vi "Log Data.vi"(0 "Test Inputs":T2 {"Nominal Output Voltage in V" format="%#.5g"; "Load Current in A" format="%#.5g"}, 5 "Test Results":T1 {"Measured Input Voltage in V" format="%#.5g"; "Dropout Voltage in V" format="%#.5g"; "Measured Output Voltage in V" format="%#.5g"}, 7 "DataLogger File Path":path, 11 "error in (no error)":errorcluster) -> (15 "error out":errorcluster)   [LabVIEW 2020, in "LDO Dropout Voltage.lvlib"]
uses:
  LDO Dropout Voltage.lvlib
  Typedefs/Test Inputs.ctl
  Typedefs/Advance Settings.ctl
  Reusables/Instrument APIs/Load Output Function.ctl
  Typedefs/Test Results.ctl
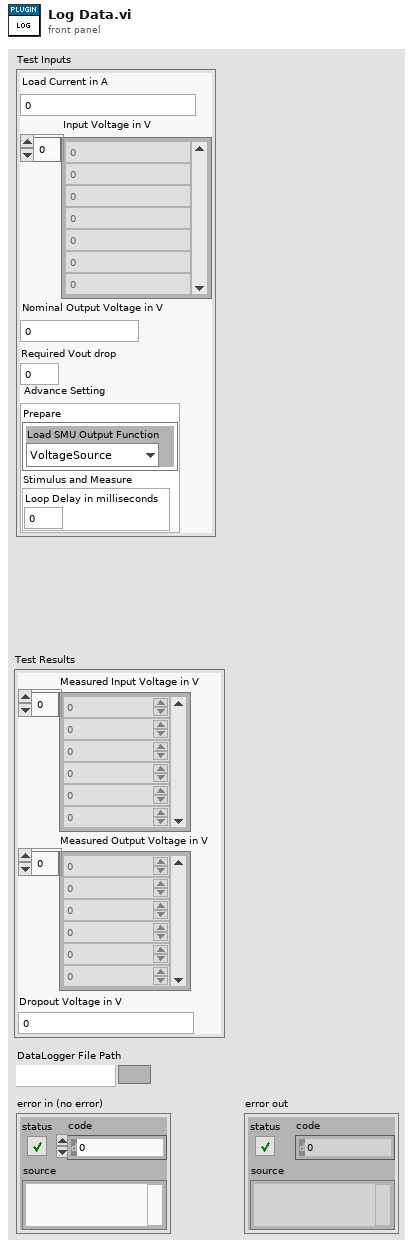
[diagram p1: front panel]
types:
  T1 = typedef "LDO Dropout Voltage.lvlib/Test Results.ctl" = cluster{"Measured Input Voltage in V":dbl[], "Measured Output Voltage in V":dbl[], "Dropout Voltage in V":dbl}
  T2 = typedef "LDO Dropout Voltage.lvlib/Test Inputs.ctl" = cluster{"Load Current in A":dbl, "Input Voltage in V":dbl[], "Nominal Output Voltage in V":dbl, "Required Vout drop":dbl, "Advance Setting":T3}
  T3 = typedef "LDO Dropout Voltage.lvlib/Advance Settings.ctl" = cluster{"Prepare":cluster{"Load SMU Output Function":T4}, "Stimulus and Measure":cluster{"Loop Delay in milliseconds":u32}}
  T4 = typedef "Load Output Function.ctl" = enum16{"VoltageSource", "CurrentSource"}
  T5 = enum16{"open", "replace", "create", "open or create", "replace or create", "replace or create with confirmation"}
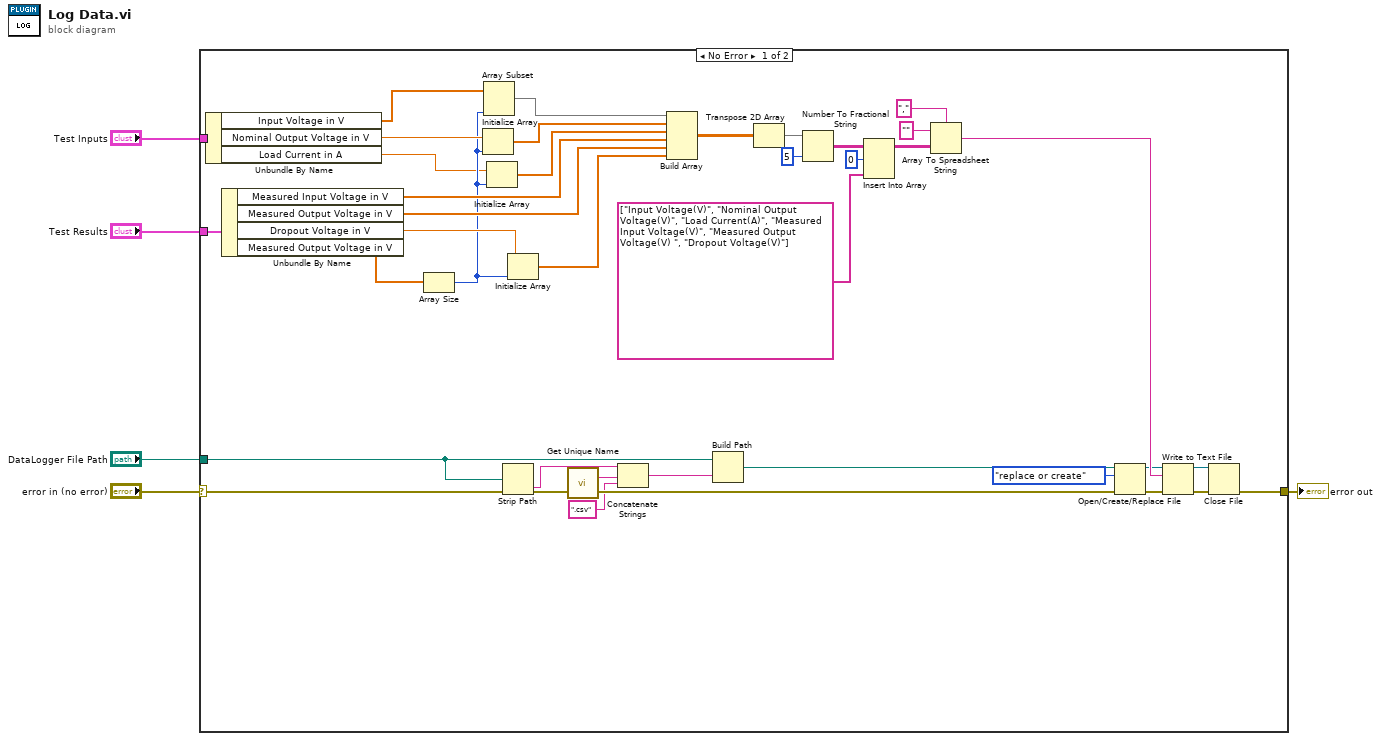
[diagram p0: block diagram]
diagram:
  n1 = case shown="No Error" "error in (no error)" {
    selector: "error in (no error)" -> [w20 w43]
    tunnel: [w28 w43] -> w4
    tunnel: "Test Inputs" -> [w42 _]
    tunnel: "Test Results" -> [w41 _]
    tunnel: "DataLogger File Path" -> [w8 _]
    frame No Error {
      n2 = Unbundle By Name(w42) -> ("Input Voltage in V"=w23:dbl[], "Nominal Output Voltage in V"=w33:dbl, "Load Current in A"=w18:dbl)
      n3 = Unbundle By Name(w41) -> ("Measured Input Voltage in V"=w38:dbl[], "Measured Output Voltage in V"=w39:dbl[], "Dropout Voltage in V"=w31:dbl, "Measured Output Voltage in V"=w29:dbl[])
      n4 = Array Size(array=w29) -> (size(s)=w19:i32)
      n5 = Initialize Array(w33, w19) -> (w32:dbl[])
      n6 = Array Subset(array=w23, length=w19) -> (w22:dbl[])  [unwired: 1 in]
      n7 = Initialize Array(w18, w19) -> (w17:dbl[])
      n8 = Strip Path(path=w8) -> (name=w10:string)  [unwired: 1 out]
      n9 = Initialize Array(w31, w19) -> (w30:dbl[])
      n10 = call "Get Unique Name.vi"() -> ("Unique String"=w11:string)  [unwired: 14 in, 1 out]
      n11 = Concatenate Strings(w10, w11, ".csv" ("format string")) -> (w7:string)
      n12 = Build Array(w22, w32, w17, w38, w39, w30) -> (w37:dbl[][])
      n13 = Build Path(base path=w8, name or relative path=w7) -> (appended path=w6:path)
      n14 = Transpose 2D Array(2D array=w37) -> (transposed array=w40:dbl[][])
      n15 = Number To Fractional String(number=w40, precision (6)=i16 5) -> (F-format string=w34:string[][])  [unwired: 2 in]
      n16 = Insert Into Array(array=w34, index (row)=0, new element=string[] ["Input Voltage(V)", "Nominal Output Voltage(V)", "Load Current(A)", "Measured Input Voltage(V)", "Measured Output Voltage(V) ", "Dropout Voltage(V)"] ("new element/subarray")) -> (w25:string[][])  [unwired: 1 in]
      n17 = Array To Spreadsheet String(delimiter (Tab)=",", array=w25, 3:"" ("format string")) -> (spreadsheet string=w24:string)
      n18 = Open/Create/Replace File(file path (use dialog)=w6, error in=w20, operation (0:open)=T5."replace or create") -> (refnum out=w14:refnum<file>, error out=w16:errorcluster)  [unwired: 3 in, 1 out]
      n19 = Write to Text File(file (use dialog)=w14, text=w24, error in=w16) -> (refnum out=w13:refnum<file>, error out=w15:errorcluster)  [unwired: 1 in, 1 out]
      n20 = Close File(refnum=w13, error in=w15) -> (error out=w28:errorcluster)  [unwired: 1 out]
    }
    frame Error {
    }
  }
  "error out" <- w4
